vi "Motor DC controlado com PWM.vi"() -> ()   [LabVIEW 2018]
uses:
  <vilib>/Waveform/WDTOps.llb/WDT Align Waveform Timestamps DBL.vi
panel:
  out "x-y":dbl
  out "thD":dbl
  out "tempo":dbl
  out "T":dbl
  out "th":dbl
  out "Sentido":enum16{"Horário", "Anti-Horário"}(ring)
  out "Duty Cycle":dbl
  in  "Tab Control":enum32{"Posição", "Velocidade", "Aceleração"}(tab)
  out "Posição Acumulada":waveform(dbl)(graph) caption="Velocidade"
  out "Velocidade Acumulada":waveform(dbl)[](graph) caption="Velocidade"
  out "Aceleração acumulada":waveform(dbl)(graph)
  in  "Zerar Rede Neural":bool
  in  "Tabela de controle":T1(tab)=enum."Controle Cossenoidal"
  in  "Posicao Angular":dbl(knob) min=-45.0 max=45.0 step=5.0 scale=-45.0..45.0
  in  "Amplitude":dbl(knob)=45.0 min=0.0 max=45.0 step=1.0 scale=0.0..45.0
  in  "Frequencia (Hz)":dbl(knob)=0.10000000000000002 min=0.0 max=3.0 step=0.1 scale=0.0..20.0
  in  "Amplitude 2":dbl(knob)=45.0 min=0.0 max=45.0 step=1.0 scale=0.0..45.0
  in  "Frequencia (Hz) 2":dbl(knob)=0.10000000000000002 min=0.0 max=3.0 step=0.1 scale=0.0..3.0
  in  "Período":dbl(knob)=2.5 min=1.5 max=10.0 step=0.5 scale=1.5..10.0
  in  "Hiperparâmetros - Rede Neural":T2={"LIMin"=15.0, "srpC"=60.0, "kIN"=20.0, "phiIN"=15.0, "apIN"=1.8, "Min"=100.0} {"Min" min=1.0 step=1.0; "apIN" min=0.0 step=0.1; "phiIN" step=0.1; "kIN" min=1.0 step=1.0; "srpC" min=1.0 step=1.0; "LIMin" min=0.0 step=0.1}
  in  "Lambda":dbl
  in  "Redução de vibração":bool
  out "Aceleração":dbl[](graph)
  out "Velocidade":dbl[][](graph)
  in  "Frequência do PWM":dbl
  in  "stop":bool
  out "Posição":dbl[](graph)
  in  "Initialize":bool
  in  "DC_Vin":dbl
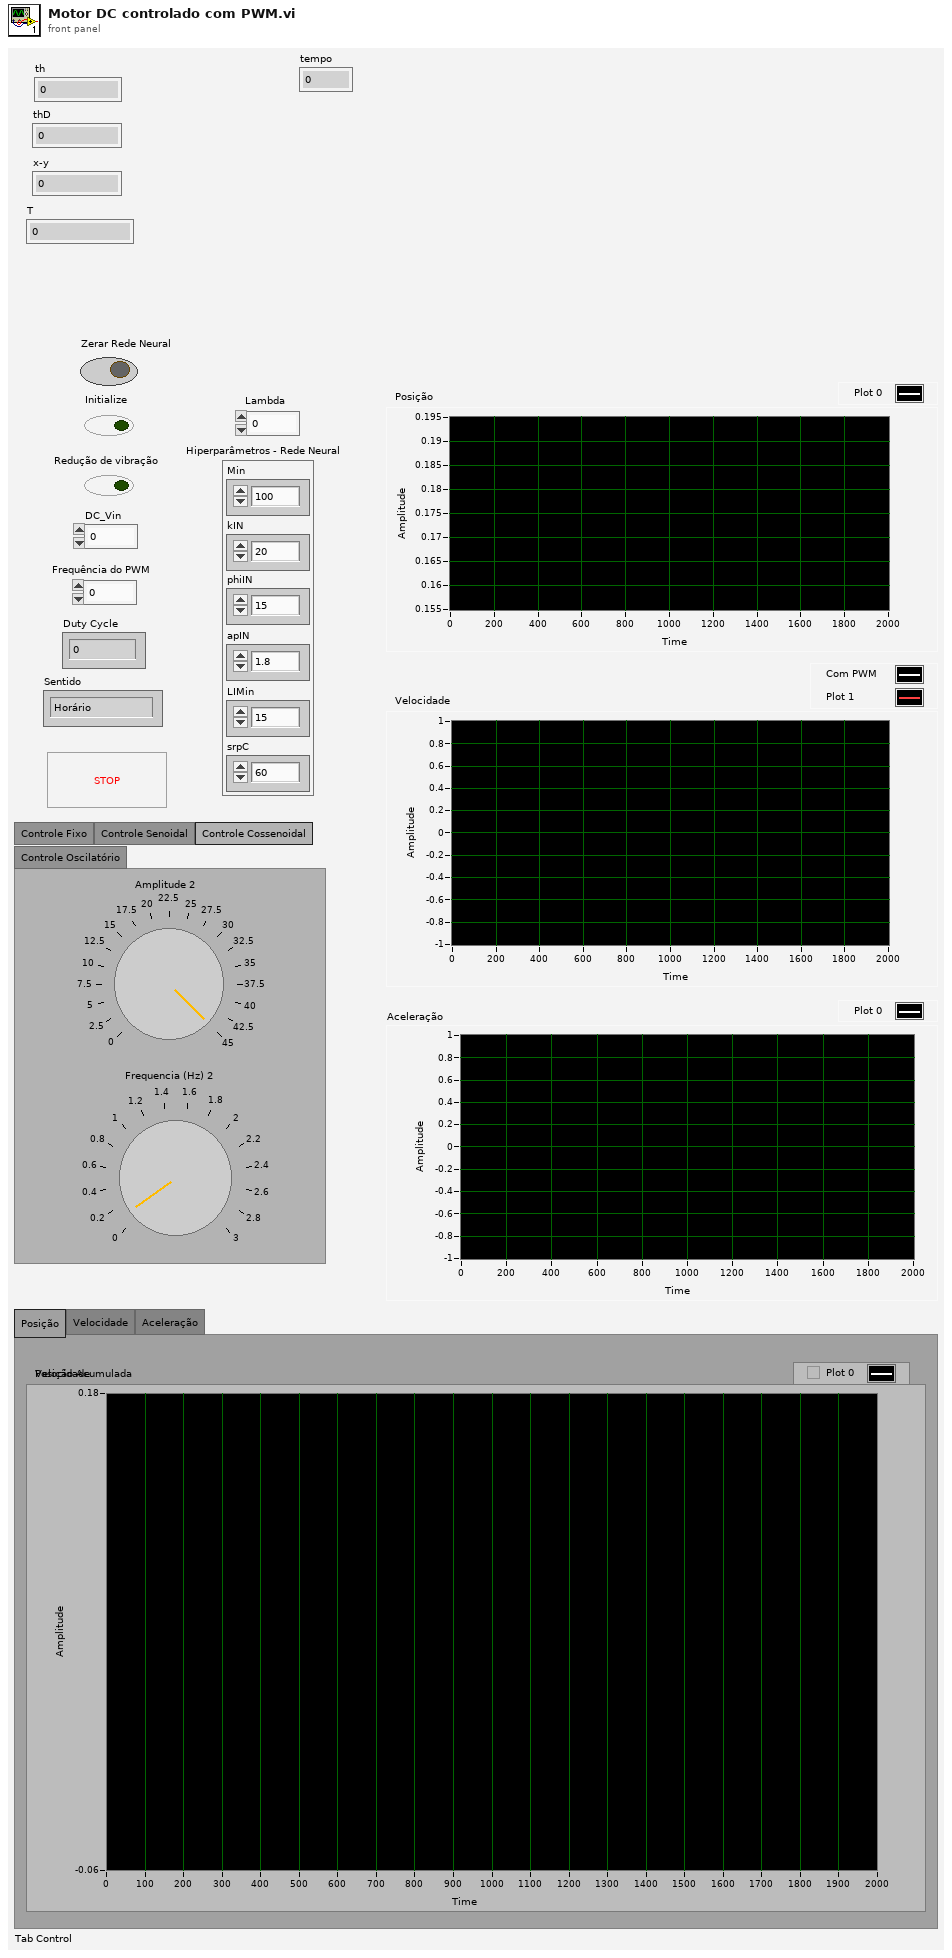
[diagram p1: front panel]
types:
  T1 = enum32{"Controle Fixo", "Controle Senoidal", "Controle Cossenoidal", "Controle Oscilatório"}
  T2 = cluster{"LIMin":dbl, "srpC":dbl, "kIN":dbl, "phiIN":dbl, "apIN":dbl, "Min":dbl}
  T3 = cluster{"thD":dbl, "thpD":dbl, "thppD":dbl, "thpppD":dbl}
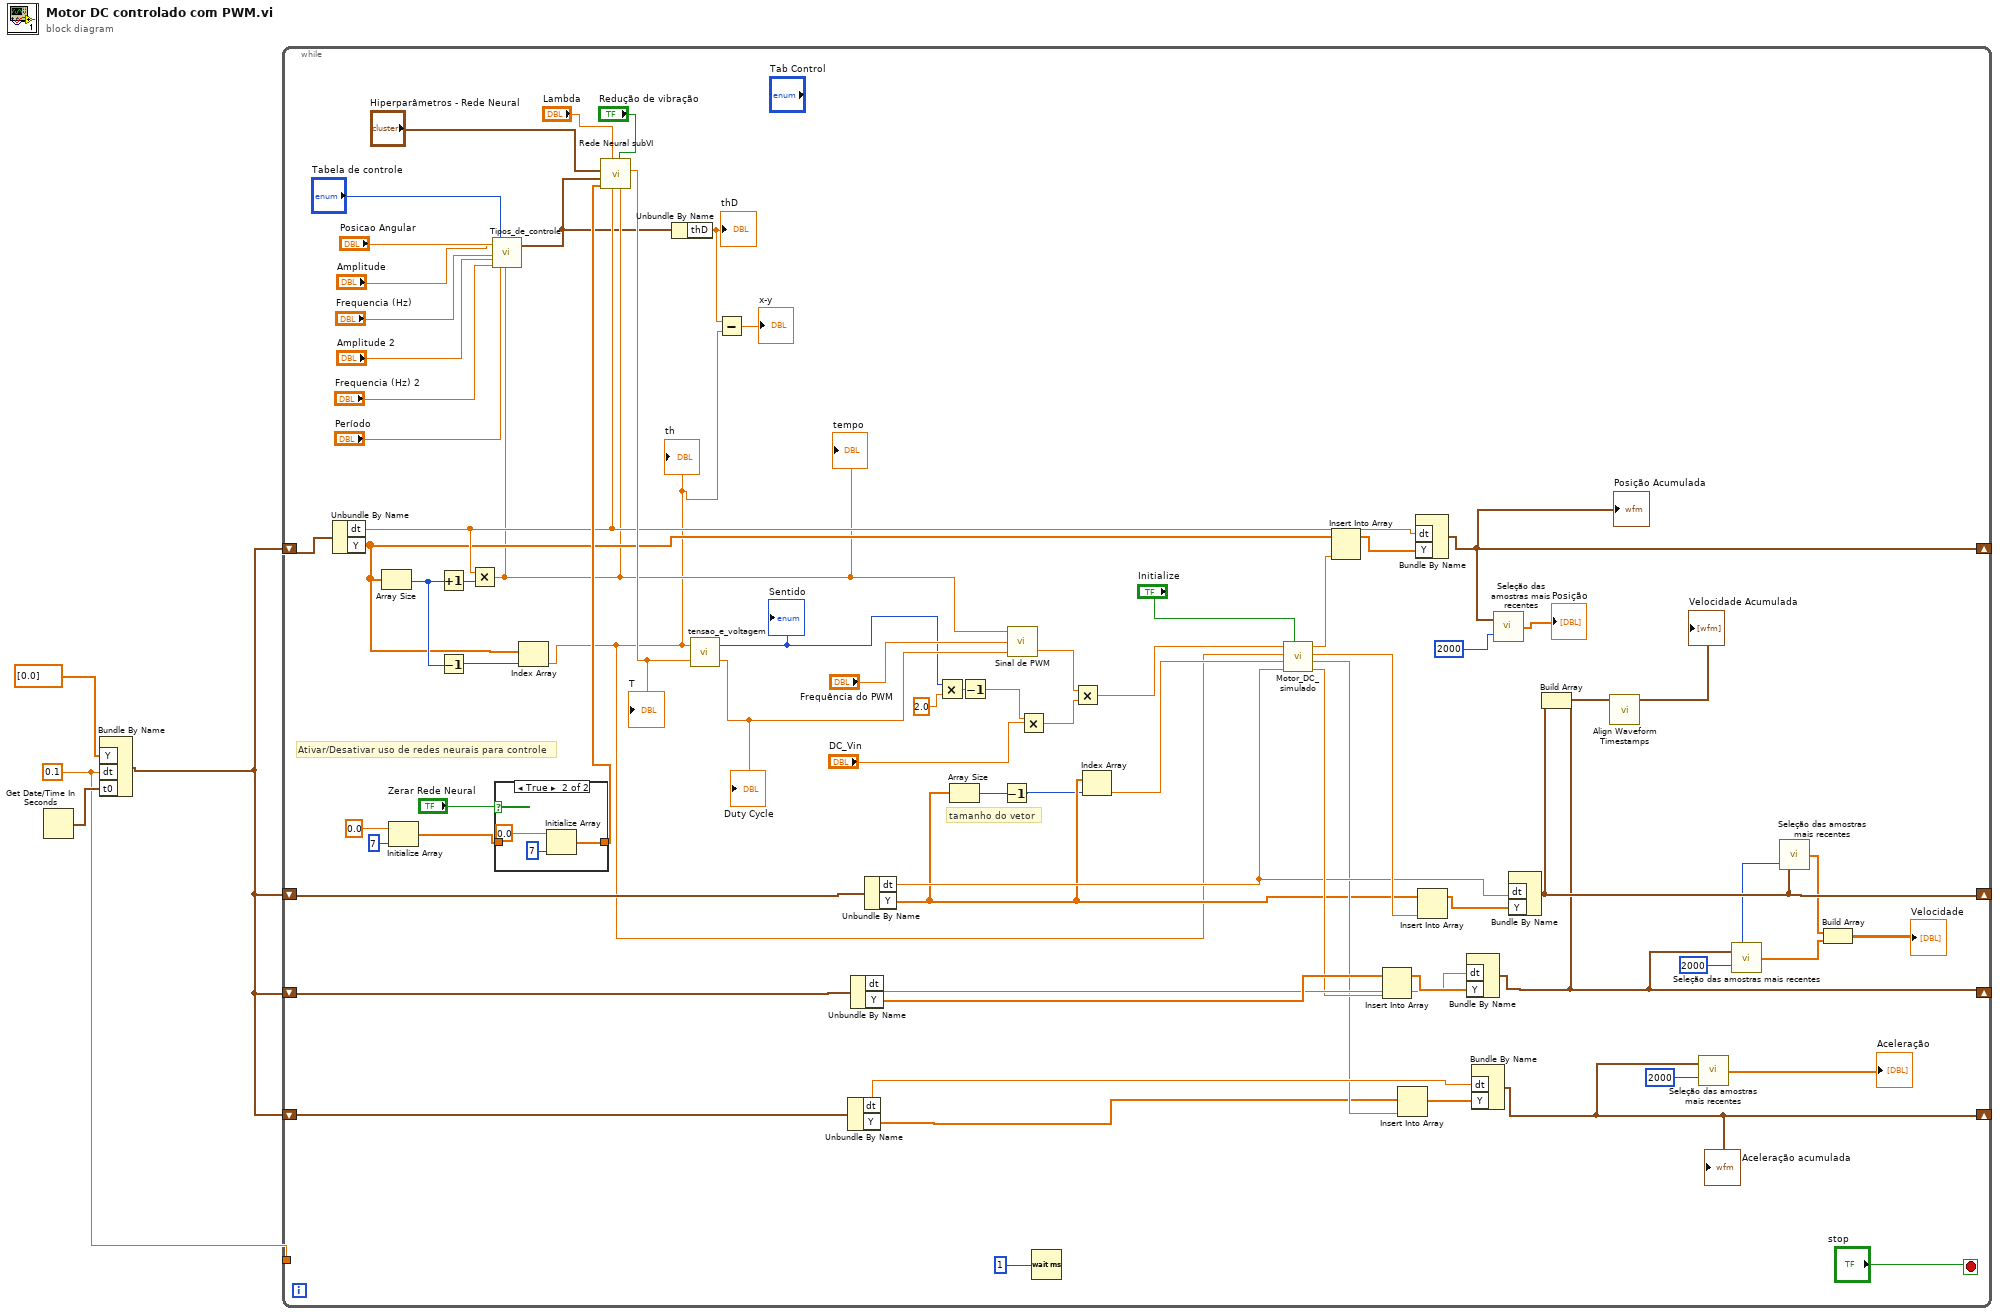
[diagram p0: block diagram]
diagram:
  w2 = 0.1 ("dt")
  n1 = Get Date/Time In Seconds() -> (seconds since 1Jan1904=w3:timestamp)
  n2 = Bundle By Name("Y"=dbl[] [0.0], "dt"=w2, "t0"=w3) -> (w1:waveform(dbl))  [unwired: 1 in]
  n3 = while {
    shift-right: [w57] -> _
    shift-left: w1 -> [w62]
    shift-right: [w56] -> _
    shift-left: w1 -> [w75]
    shift-right: [w55] -> _
    shift-left: w1 -> [w71]
    tunnel: w2 -> [_]
    shift-right: [w38] -> _
    shift-left: w1 -> [w41]
    stop <- "stop" stop-if-true
    w51 = 2000 ("Número de amostras no gráfico 2")
    # "Ativar/Desativar uso de redes neurais para controle"
    # "tamanho do vetor"
    n4 = Unbundle By Name(w62) -> ("dt"=w18:dbl, "Y"=w15:dbl[])
    n5 = Array Size(array=w15) -> (size(s)=w16:i32)
    n6 = Initialize Array(0.0 ("element"), 7 ("dimension size")) -> (w31:dbl[])
    n7 = Increment(x=w16) -> (x+1=w61:i32)
    n8 = Decrement(x=w16) -> (x-1=w17:i32)
    n9 = Multiply(x=w18, y=w61) -> (x*y=w12:dbl)
    "tempo" <- w12
    n10 = call "Tipos_de_controle.vi"("Posicao Angular"="Posicao Angular", "Amplitude"="Amplitude", "Frequencia (Hz)"="Frequencia (Hz)", "Amplitude 2"="Amplitude 2", "Frequencia (Hz) 2"="Frequencia (Hz) 2", "Tabela de controle"="Tabela de controle", "Período"="Período", "Tempo"=w12) -> ("Valores desejados"=w11:T3)  [unwired: 11 in]
    n11 = case shown="True" "Zerar Rede Neural" {
      tunnel: [w79 w80] -> w20
      tunnel: w31 -> [w79 _]
      frame False {
      }
      frame True {
        n12 = Initialize Array(0.0 ("element"), 7 ("dimension size")) -> (w80:dbl[])
      }
    }
    n13 = Index Array(array=w15, index=w17) -> (element=w7:dbl)
    "th" <- w7
    n14 = call "Rede Neural subVI.vi"("Elapsed Time (s)"=w12, "Redução de vibração"="Redução de vibração", "dt"=w18, "Lambda"="Lambda", "w"=w20, "Valores atuais"=w11, "Hiperparâmetros - Rede Neural"="Hiperparâmetros - Rede Neural") -> ("T"=w21:dbl)  [unwired: 4 in]
    "T" <- w21
    n15 = Unbundle By Name(w11) -> ("thD"=w10:dbl)
    "thD" <- w10
    n16 = call "tensao_e_voltagem.vi"("T"=w21, "th"=w7) -> ("Duty Cycle"=w14:dbl, "Sentido"=w13:enum16{"Horário", "Anti-Horário"})
    "Duty Cycle" <- w14
    "Sentido" <- w13
    n17 = Subtract(x=w10, y=w7) -> (x-y=→"x-y":dbl)
    n18 = Unbundle By Name(w41) -> ("dt"=w42:dbl, "Y"=w36:dbl[])
    n19 = Unbundle By Name(w71) -> ("dt"=w72:dbl, "Y"=w74:dbl[])
    n20 = Unbundle By Name(w75) -> ("dt"=w45:dbl, "Y"=w35:dbl[])
    n21 = Multiply(x=w13, y=2.0) -> (x*y=w49:dbl)
    n22 = Array Size(array=w35) -> (size(s)=w34:i32)
    n23 = Decrement(x=w49) -> (x-1=w47:dbl)
    n24 = Decrement(x=w34) -> (x-1=w33:i32)
    n25 = call "Sinal de PWM.vi"("duty cycle"=w14, "Frequência do PWM"="Frequência do PWM", "Tempo atual"=w12) -> ("Resultado numérico"=w64:dbl)  [unwired: 1 out]
    n26 = Multiply(x=w47, y="DC_Vin") -> (x*y=w46:dbl)
    n27 = Wait (ms)(milliseconds to wait=u32 1 ("y")) -> ()  [unwired: 1 out]
    n28 = Multiply(x=w64, y=w46) -> (x*y=w63:dbl)
    n29 = Index Array(array=w35, index=w33) -> (element=w44:dbl)
    n30 = call "Motor_DC_simulado.vi"("Initialize"="Initialize", "dt"=w45, "Velocidade anterior"=w44, "Posiçao anterior"=w7, "DC_Vin"=w63) -> ("Tensão fornecida ao motor"=w68:dbl, "Aceleração"=w40:dbl, "Velocidade"=w67:dbl, "Posição"=w66:dbl)  [unwired: 2 in]
    n31 = Insert Into Array(array=w15, new element=w66) -> (w77:dbl[])  [unwired: 1 in]
    n32 = Insert Into Array(array=w74, new element=w68) -> (w73:dbl[])  [unwired: 1 in]
    n33 = Insert Into Array(array=w36, new element=w40) -> (w43:dbl[])  [unwired: 1 in]
    n34 = Bundle By Name("dt"=w18, "Y"=w77) -> (w57:waveform(dbl))  [unwired: 1 in]
    "Posição Acumulada" <- w57
    n35 = Insert Into Array(array=w35, new element=w67) -> (w76:dbl[])  [unwired: 1 in]
    n36 = Bundle By Name("dt"=w72, "Y"=w73) -> (w55:waveform(dbl))  [unwired: 1 in]
    n37 = Bundle By Name("dt"=w42, "Y"=w43) -> (w38:waveform(dbl))  [unwired: 1 in]
    "Aceleração acumulada" <- w38
    n38 = call "Seleção das amostras mais recentes.vi"("Número de amostras no gráfico"=2000, "Vetor de entrada"=w57) -> ("Amostras do gráfico"=→"Posição":dbl[])
    n39 = Bundle By Name("dt"=w45, "Y"=w76) -> (w56:waveform(dbl))  [unwired: 1 in]
    n40 = Build Array "Build Array"(w56, w55) -> (w70:waveform(dbl)[])
    n41 = call-poly <vilib>:"Align Waveform Timestamps.vi"("waveforms in"=w70) -> ("waveforms out"=→"Velocidade Acumulada":waveform(dbl)[])  [unwired: 9 in, 1 out]
    n42 = call "Seleção das amostras mais recentes.vi"("Número de amostras no gráfico"=2000 ("Número de amostras no gráfico 2"), "Vetor de entrada"=w38) -> ("Amostras do gráfico"=→"Aceleração":dbl[])
    n43 = call "Seleção das amostras mais recentes.vi"("Número de amostras no gráfico"=w51, "Vetor de entrada"=w55) -> ("Amostras do gráfico"=w54:dbl[])
    n44 = call "Seleção das amostras mais recentes.vi"("Número de amostras no gráfico"=w51, "Vetor de entrada"=w56) -> ("Amostras do gráfico"=w53:dbl[])
    n45 = Build Array "Build Array"(w53, w54) -> (→"Velocidade":dbl[][])
  }
